vi "raddrizzatore.vi"(1 "bipolare (true)":bool, 2 "waveform":waveform(dbl)) -> (0 "output waveform":waveform(dbl))   [LabVIEW 2009]
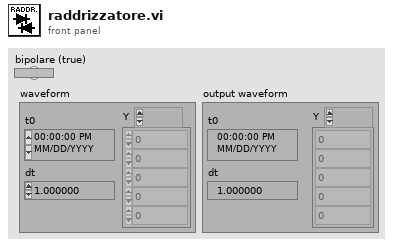
[diagram p1: front panel]
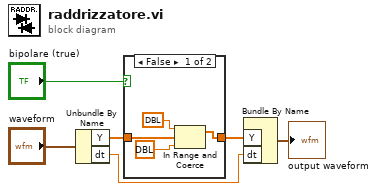
[diagram p0: block diagram]
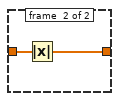
[diagram p2: hidden frame]
diagram:
  n1 = Unbundle By Name("waveform") -> ("Y"=w4:dbl[], "dt"=w2:dbl)
  n2 = case shown="False" "bipolare (true)" {
    tunnel: w4 -> [w8 w12]
    tunnel: [w7 w11] -> w3
    frame #0 {
      n3 = In Range and Coerce(upper limit=dbl ?, x=w8, lower limit=dbl ?) -> (coerced(x)=w7:dbl[])  [unwired: 1 out]
    }
    frame #1 {
      n4 = Absolute Value(x=w12) -> (abs(x)=w11:dbl[])
    }
  }
  n5 = Bundle By Name("Y"=w3, "dt"=w2) -> (→"output waveform":waveform(dbl))  [unwired: 1 in]
